vi "NotOfValues.vi"(8 "error in (no error)":errorcluster, 10 "Inputdata":dbl[](array[numeric])) -> (0 "error out":errorcluster, 3 "Outputvalues":dbl[](array[numeric]))   [LabVIEW 2019, in "Zen Analytics.lvlib" / "Zen Analytics.lvclass"]
uses:
  Zen Analytics.lvclass
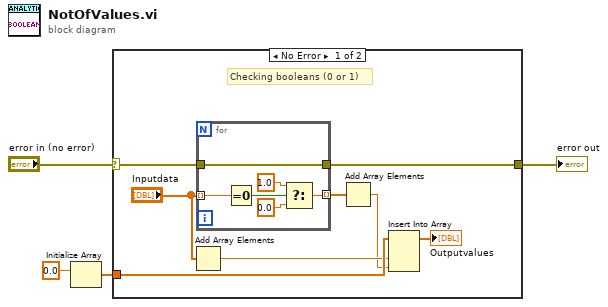
[diagram p0: block diagram]
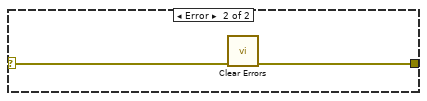
[diagram p2: hidden frame]
diagram:
  n1 = Initialize Array(0.0 ("element")) -> (w2:dbl[])  [unwired: 1 in]
  n2 = case shown="No Error" "error in (no error)" {
    selector: "error in (no error)" -> [w11 w20]
    tunnel: [w12 w19] -> w1
    tunnel: w2 -> [w8 _]
    frame No Error {
      # "Checking booleans (0 or 1)"
      n3 = Add Array Elements(numeric array="Inputdata") -> (sum=w7:dbl)
      n4 = for {
        tunnel: "Inputdata" -> [w18] mode=indexing
        tunnel: [w14] -> w9 mode=indexing
        tunnel: [w13] -> w12
        tunnel: w11 -> [w13]
        n5 = Equal To 0?(x=w18) -> (x = 0?=w17:bool)
        n6 = Select(t=1.0, s=w17, f=0.0) -> (s? t:f=w14:dbl)
      }
      n7 = Add Array Elements(numeric array=w9) -> (sum=w6:dbl)
      n8 = Insert Into Array(array=w8, new element #1=w7, new element #2=w6) -> (→"Outputvalues":dbl[])  [unwired: 1 in]
    }
    frame Error {
      n9 = call <vilib>:"Clear Errors.vi"("error in (no error)"=w20) -> ("error out"=w19:errorcluster)  [unwired: 5 in, 1 out]
    }
  }
  "error out" <- w1
